vi "get major and minor version string.vi"(11 "full version":string) -> (3 "major.minor version":string)   [LabVIEW 2013, in "TBM configuration.lvclass"]
doc: "Strips any version information after the major and minor version numbers. This is intended to be used by <b>from string.vi</b>, as data changes should result in a major or minor version number change."
uses:
  TBM configuration.lvclass
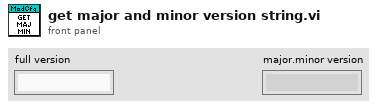
[diagram p1: front panel]
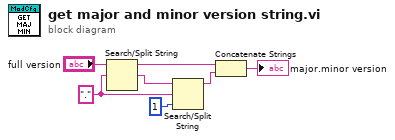
[diagram p0: block diagram]
diagram:
  w3 = "." ("search string/char (-)")
  n1 = Search/Split String(string="full version", search string/char (-)=w3) -> (substring before match=w5:string, match + rest of string=w6:string)  [unwired: 1 in, 1 out]
  n2 = Search/Split String(string=w6, search string/char (-)=w3, offset (0)=1) -> (substring before match=w4:string)  [unwired: 2 out]
  n3 = Concatenate Strings(w5, w4) -> (→"major.minor version":string)
